vi "LabVIEW NPOI.vi"   [LabVIEW 2017]
uses:
  <vilib>/Platform/browser.llb/Open URL in Default Browser (path).vi
panel:
  # "Opening LabVIEW NPOI Help..."
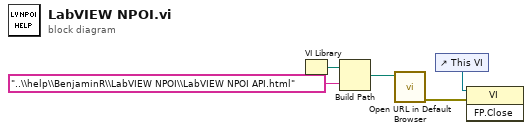
[diagram p0: block diagram]
diagram:
  n1 = VI Library() -> (path=w3:path)
  n2 = Build Path(base path=w3, name or relative path="..\\help\\BenjaminR\\LabVIEW NPOI\\LabVIEW NPOI API.html" ("URL")) -> (appended path=w2:path)
  n3 = call-poly <vilib>:"Open URL in Default Browser.vi"("path"=w2) -> ("error out"=w5:errorcluster)  [unwired: 5 in, 1 out]
  n4 = control-ref of="This VI"() -> (w4:refnum<vi>)
  n5 = invoke class="VI" method="FP.Close"(reference=w4, error in=w5) -> ()  [unwired: 1 in, 3 out]
